vi "MagnitudeFFT (SubVI).vi"(11 "Windowed Signal Array":dbl[](array[numeric])) -> (3 "Magnitude FFT":dbl[](array[numeric]))   [LabVIEW 2015]
uses:
  <vilib>/Analysis/2dsp.llb/Real FFT.vi
  <vilib>/Analysis/NI_AALPro.lvlib
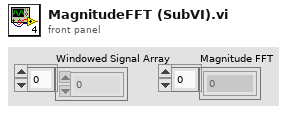
[diagram p1: front panel]
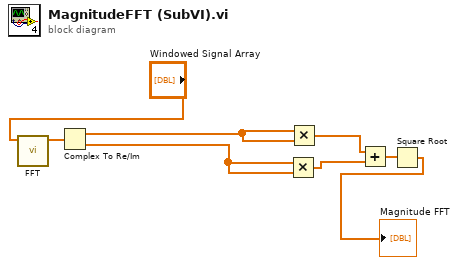
[diagram p0: block diagram]
diagram:
  n1 = call-poly <vilib>:"FFT.vi"("X"="Windowed Signal Array") -> ("FFT {X}"=w1:cdb[])  [unwired: 9 in, 1 out]
  n2 = Complex To Re/Im(x + iy=w1) -> (x=w3:dbl[], y=w2:dbl[])
  n3 = Multiply(x=w2, y=w2) -> (x*y=w5:dbl[])
  n4 = Multiply(x=w3, y=w3) -> (x*y=w4:dbl[])
  n5 = Add(x=w4, y=w5) -> (x+y=w6:dbl[])
  n6 = Square Root(x=w6) -> (sqrt(x)=→"Magnitude FFT":dbl[])
